vi "Command_Puke_Op.vi"(0 "Startup":bool, 1 "Puke_Op_Goal_Velocity":dbl=1000.0 format="%#_13g", 2 "Timeout":dbl, 3 "Puke_Op_Cowl_Angle":dbl=61.0 format="%#_13g") -> (6 "Reint":bool, 7 "Completed":bool, 8 "Puke_Op_Goal_Velocity":dbl, 9 "Puke_Op_Cowl_Angle":dbl)   [LabVIEW 2020]
uses:
  Auto Utilities/Command_Execution_State.ctl
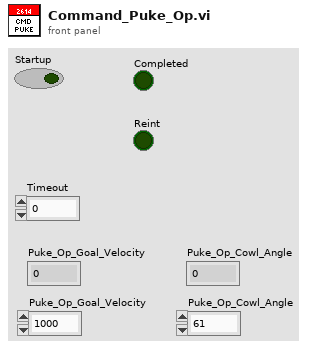
[diagram p1: front panel]
types:
  T1 = typedef "Command_Execution_State.ctl" = enum16{"Initialize", "Execute", "Finish"}
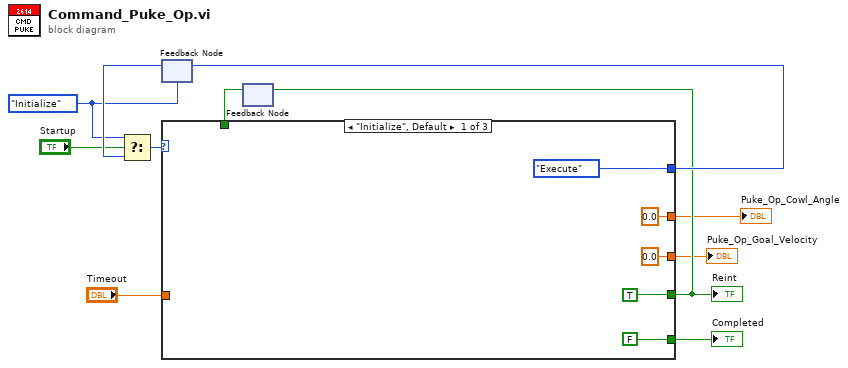
[diagram p0: block diagram]
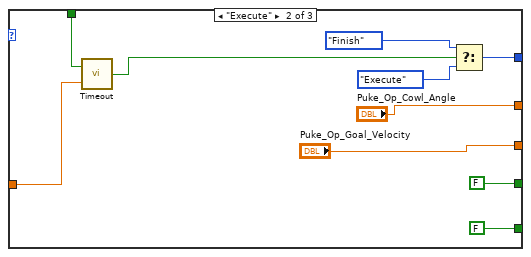
[diagram p2: hidden frame]
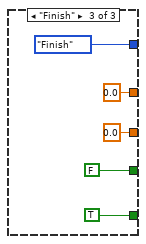
[diagram p3: hidden frame]
diagram:
  w6 = Command_Execution_State."Initialize" ("Play State")
  n1 = feedback #1(w6) -> (w9:T1)
  n2 = Select(t=w6, s="Startup", f=w9) -> (s? t:f=w11:T1)
  n3 = feedback #2() -> (w5:bool)  [unwired: 1 in]
  n4 = case shown="\"Initialize\", Default" w11 {
    tunnel: [Command_Execution_State."Execute" ("Play State") w22 Command_Execution_State."Finish" ("Play State")] -> w10
    tunnel: [FALSE FALSE TRUE] -> w8
    tunnel: [TRUE FALSE FALSE] -> w3
    tunnel: w5 -> [_ w24 _]
    tunnel: "Timeout" -> [_ w23 _]
    tunnel: [0.0 ("Puke_Op_Goal_Velocity") "Puke_Op_Goal_Velocity" 0.0 ("Puke_Op_Goal_Velocity")] -> w2
    tunnel: [0.0 ("Puke_Op_Cowl_Angle") "Puke_Op_Cowl_Angle" 0.0 ("Puke_Op_Cowl_Angle")] -> w1
    frame "Initialize", Default {
    }
    frame "Execute" {
      n5 = call "Timeout.vi"("Timeout"=w23, "Initialize"=w24) -> ("Timed Out?"=w19:bool)
      n6 = Select(t=Command_Execution_State."Finish" ("Play State"), s=w19, f=Command_Execution_State."Execute" ("Play State")) -> (s? t:f=w22:T1)
    }
    frame "Finish" {
    }
  }
  "Completed" <- w8
  "Reint" <- w3
  "Puke_Op_Goal_Velocity" <- w2
  "Puke_Op_Cowl_Angle" <- w1
  n7 = feedback-in #1(w10) -> ()
  n8 = feedback-in #2(w3) -> ()
